vi "Fault Detection with Pattern Recognition.vi"() -> ()   [LabVIEW 2023]
doc: "This example shows the application of autoregressive (AR) modeling in fault detection with pattern recognition.\n\nFault diagnosis of industrial equipment can be performed with pattern recognition. You usually build an AR or autoregressive-moving average (ARMA) model for a signal (pressure, temperature, vibration etc.) that the equipment generates and use the model coefficients to form a judgment pattern criterion to diagnose the equipment. \n\nPattern recognition is performed in the following steps:\n1) Find the patterns that indicate the equipment is in good state and the patterns that indicate bad state.\n2) Compare the current pattern of the equipment with known patterns to find out if current equipment is in bad state.\n\nIn this example, the coefficients of a two-order AR model are used as the judgment pattern. Different system state belongs to different zones on an XY graph with the first and the second AR coefficient being the x-axis and the y-axis, respectively.\n\nThis example uses the TSA AR Modeling VI to build the AR model for the signal.\n\n<b>Instructions:</b>\nRun this VI. Observe when the fault occurs."
uses:
  <vilib>/Analysis/baseanly.llb/Mean (DBL).vi
  <vilib>/addons/Time Series Analysis/Modeling and Prediction.llb/TSA AR Modeling (Array).vi
  <vilib>/addons/_Advanced Signal Processing/NI_AdvSigProcTSA.lvlib
  <vilib>/Analysis/NI_AALBase.lvlib
panel:
  out "aspt-left-top":bool
  in  "stop":bool
  out "Current mode":cluster{"AR (1)":dbl, "AR (2)":dbl}={"AR (1)"=1.1774883983885933, "AR (2)"=0.8725048676880719} {"AR (2)" format="%#_2g"; "AR (1)" format="%#_2g"}
  out "Simulated Time Series":dbl[](graph)
  in  "Threshold":dbl=0.2 min=1e-09
  out "Fault Mode?":bool
  out "Current System State":cluster{dbl, dbl}[](graph)
  out "Fault mode mean":cluster{"AR (1)":dbl, "AR (2)":dbl}={"AR (1)"=1.1774883983885933, "AR (2)"=0.8725048676880719} {"AR (2)" format="%#_2g"; "AR (1)" format="%#_2g"}
  out "Normal mode mean":cluster{"AR (1)":dbl, "AR (2)":dbl}={"AR (1)"=0.494671953835734, "AR (2)"=0.7033327545625112} {"AR (2)" format="%#_2g"; "AR (1)" format="%#_2g"}
  out "System State Statistics":cluster{dbl[], dbl[]}[](graph)
  # "Overview: Shows the application of autoregressive (AR) modeling in fault detection with pattern recognition.\nRequirements: LabVIEW Full Development System, Advanced Signal Processing Toolkit\nInstructions: \n1. Run this VI. Observe when the fault occurs.\n2. Click Stop to stop the VI."
  # "Pattern Learning"
  # "Pattern Matching (Monitoring)"
  # "Fault Mode"
  # "Fault Mode"
  # "Normal Mode"
  # "Normal Mode"
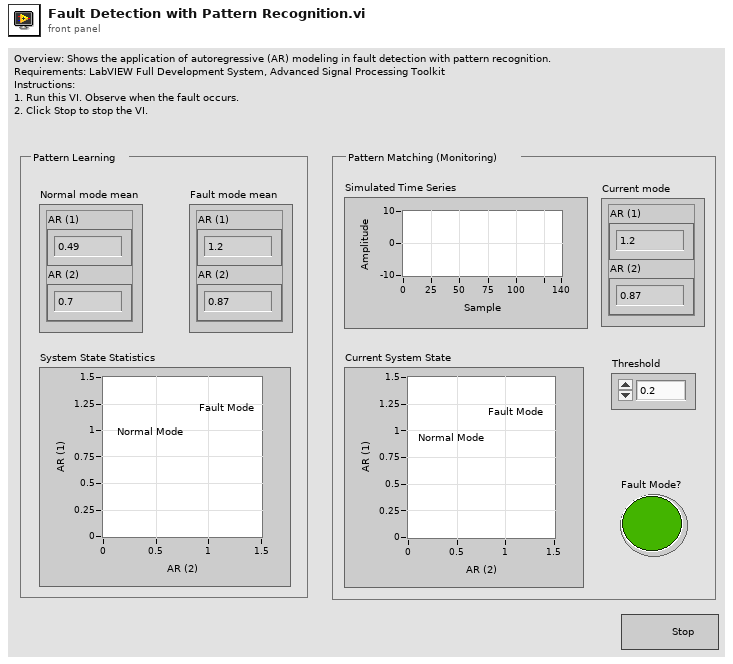
[diagram p1: front panel]
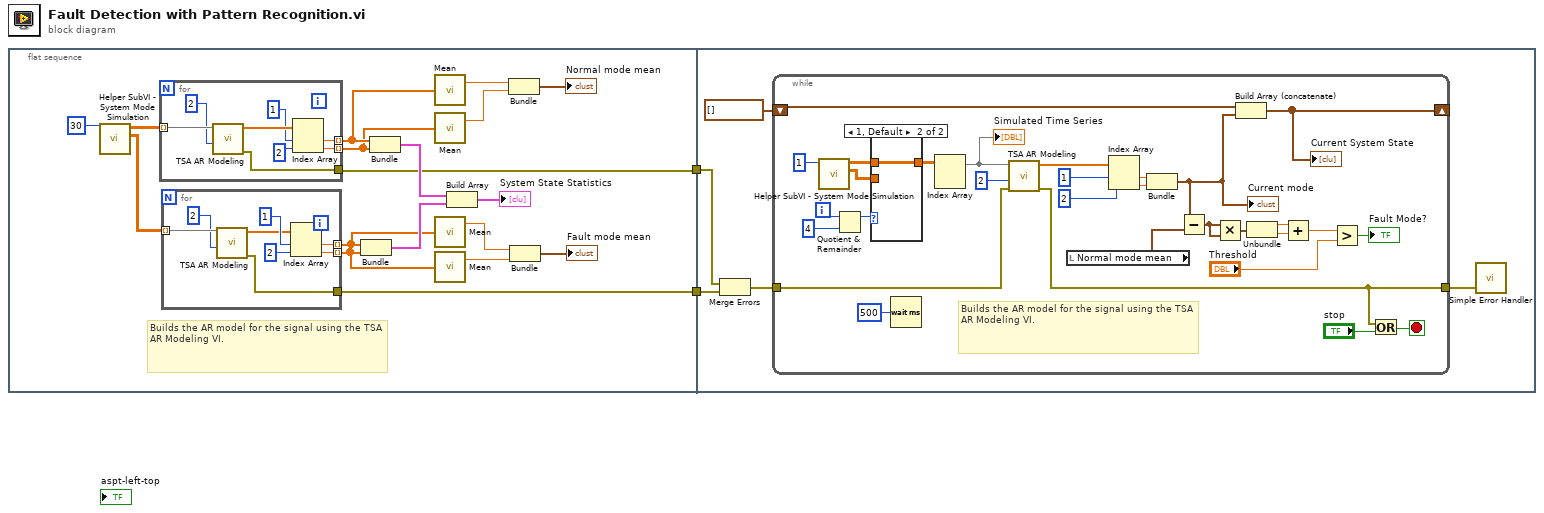
[diagram p0: block diagram]
diagram:
  n1 = flat-sequence {
    tunnel: [w7] -> w2
    tunnel: [w6] -> w1
    tunnel: w2 -> [w40]
    tunnel: w1 -> [w39]
    frame #0 {
      # "Builds the AR model for the signal using the TSA AR Modeling VI."
      n2 = call "Helper SubVI - System Mode Simulation.vi"("mode num"=30 ("Statistic num")) -> ("fault mode"=w4:dbl[][], "normal mode"=w5:dbl[][])  [unwired: 9 in]
      n3 = for {
        tunnel: w5 -> [w36] mode=indexing
        tunnel: [w31] -> w17 mode=indexing
        tunnel: [w30] -> w16 mode=indexing
        tunnel: [w29] -> w7
        n4 = call-poly <vilib>:"TSA AR Modeling.vi"("AR order"=2, "Xt"=w36) -> ("error out"=w29:errorcluster, "AR coefficients"=w34:dbl[])  [unwired: 2 in, 6 out]
        n5 = Index Array(array=w34, index #1=1 ("index"), index #2=2 ("index")) -> (element #1=w31:dbl, element #2=w30:dbl)
      }
      n6 = for {
        tunnel: w4 -> [w28] mode=indexing
        tunnel: [w23] -> w15 mode=indexing
        tunnel: [w22] -> w14 mode=indexing
        tunnel: [w21] -> w6
        n7 = call-poly <vilib>:"TSA AR Modeling.vi"("AR order"=2, "Xt"=w28) -> ("error out"=w21:errorcluster, "AR coefficients"=w24:dbl[])  [unwired: 2 in, 6 out]
        n8 = Index Array(array=w24, index #1=1 ("index"), index #2=2 ("index")) -> (element #1=w23:dbl, element #2=w22:dbl)
      }
      n9 = Bundle(w15, w14) -> (w18:cluster{dbl[], dbl[]})  [unwired: 1 out]
      n10 = Bundle(w17, w16) -> (w19:cluster{dbl[], dbl[]})  [unwired: 1 out]
      n11 = call-poly <vilib>:"Mean.vi"("X"=w17) -> ("mean"=w13:dbl)  [unwired: 1 out]
      n12 = call-poly <vilib>:"Mean.vi"("X"=w16) -> ("mean"=w12:dbl)  [unwired: 1 out]
      n13 = call-poly <vilib>:"Mean.vi"("X"=w15) -> ("mean"=w9:dbl)  [unwired: 1 out]
      n14 = call-poly <vilib>:"Mean.vi"("X"=w14) -> ("mean"=w8:dbl)  [unwired: 1 out]
      n15 = Build Array(w19, w18) -> (→"System State Statistics":cluster{dbl[], dbl[]}[])
      n16 = Bundle("mean"=w13, "mean"=w12) -> (→"Normal mode mean":cluster{"mean":dbl, "mean":dbl})  [unwired: 1 out]
      n17 = Bundle("mean"=w9, "mean"=w8) -> (→"Fault mode mean":cluster{"mean":dbl, "mean":dbl})  [unwired: 1 out]
    }
    frame #1 {
      n18 = Merge Errors(w40, w39) -> (w38:errorcluster)
      n19 = while {
        shift-right: [w58] -> _
        shift-left: cluster{dbl, dbl}[] [] -> [w59]
        tunnel: w38 -> [w49]
        tunnel: [w46] -> w37
        i -> [w71]
        stop <- w47 stop-if-true
        # "Builds the AR model for the signal using the TSA AR Modeling VI."
        n20 = call "Helper SubVI - System Mode Simulation.vi"("mode num"=1) -> ("fault mode"=w43:dbl[][], "normal mode"=w44:dbl[][])  [unwired: 9 in]
        n21 = Quotient & Remainder(x=w71, y=4) -> (x-y*floor(x/y)=w69:i32)  [unwired: 1 out]
        n22 = case shown="1, Default" w69 {
          tunnel: w44 -> [_ w73]
          tunnel: [w72 w73] -> w62
          tunnel: w43 -> [w72 _]
          frame 0 {
          }
          frame 1, Default {
          }
        }
        n23 = Wait (ms)(milliseconds to wait=u32 500 ("millisecond multiple")) -> ()  [unwired: 1 out]
        n24 = Index Array(array=w62) -> (element=w45:dbl[])  [unwired: 2 in]
        "Simulated Time Series" <- w45
        n25 = call-poly <vilib>:"TSA AR Modeling.vi"("error in (no error)"=w49, "AR order"=2, "Xt"=w45) -> ("error out"=w46:errorcluster, "AR coefficients"=w65:dbl[])  [unwired: 1 in, 6 out]
        n26 = local read "Normal mode mean"() -> (w60:cluster{"AR (1)":dbl, "AR (2)":dbl})
        n27 = Index Array(array=w65, index #1=1 ("index"), index #2=2 ("index")) -> (element #1=w61:dbl, element #2=w68:dbl)
        n28 = Bundle(w61, w68) -> (w50:cluster{dbl, dbl})  [unwired: 1 out]
        "Current mode" <- w50
        n29 = Subtract(x=w50, y=w60) -> (x-y=w57:cluster{dbl, dbl})
        n30 = Multiply(x=w57, y=w57) -> (x*y=w56:cluster{dbl, dbl})
        n31 = Build Array (concatenate)(w59, w50) -> (w58:cluster{dbl, dbl}[])
        "Current System State" <- w58
        n32 = Unbundle(w56) -> (w55:dbl, w54:dbl)
        n33 = Add(x=w55, y=w54) -> (x+y=w53:dbl)
        n34 = Greater?(x=w53, y="Threshold") -> (0:→"Fault Mode?":bool)
        n35 = Or(x=w46, y="stop") -> (x .or. y?=w47:bool)
      }
      n36 = call <vilib>:"Simple Error Handler.vi"("error in (no error)"=w37) -> ()  [unwired: 4 in, 5 out]
    }
  }
